vi "Linspace.vi"(9 "n":dbl, 10 "End":dbl, 11 "Start":dbl) -> (3 "Array":dbl[](array[numeric]))   [LabVIEW 2015]
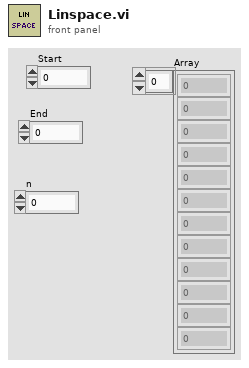
[diagram p1: front panel]
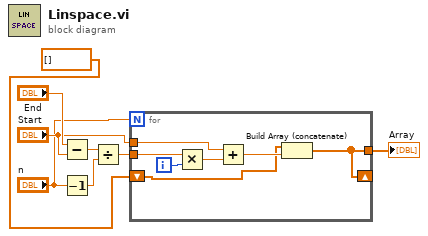
[diagram p0: block diagram]
diagram:
  n1 = Subtract(x="End", y="Start") -> (x-y=w7:dbl)
  n2 = Decrement(x="n") -> (x-1=w2:dbl)
  n3 = Divide(x=w7, y=w2) -> (x/y=w6:dbl)
  n4 = for {
    N: "n" -> [_]
    tunnel: w6 -> [w13]
    tunnel: [w9] -> w5
    tunnel: "Start" -> [w11]
    shift-right: [w9] -> _
    shift-left: dbl[] [] -> [w10]
    i -> [w14]
    n5 = Multiply(x=w13, y=w14) -> (x*y=w12:dbl)
    n6 = Add(x=w11, y=w12) -> (x+y=w15:dbl)
    n7 = Build Array (concatenate)(w10, w15) -> (w9:dbl[])
  }
  "Array" <- w5
